vi "prelim_per_setup.vi"(8 "error in":errorcluster, 11 "reference cluster":T1) -> (0 "error out":errorcluster, 3 "reference cluster":T1)   [LabVIEW 2016]
uses:
  Type Definitions/reference_cluster.ctl
  Type Definitions/vars_settings.ctl
  Type Definitions/stim_type.ctl
  Type Definitions/backlight_type.ctl
  Type Definitions/vars_runtime.ctl
  Type Definitions/data.ctl
  Type Definitions/notifier_elements_GUI.ctl
  Type Definitions/notifier_elements_DAQ.ctl
  Type Definitions/notifier_elements_write.ctl
  Type Definitions/control_references.ctl
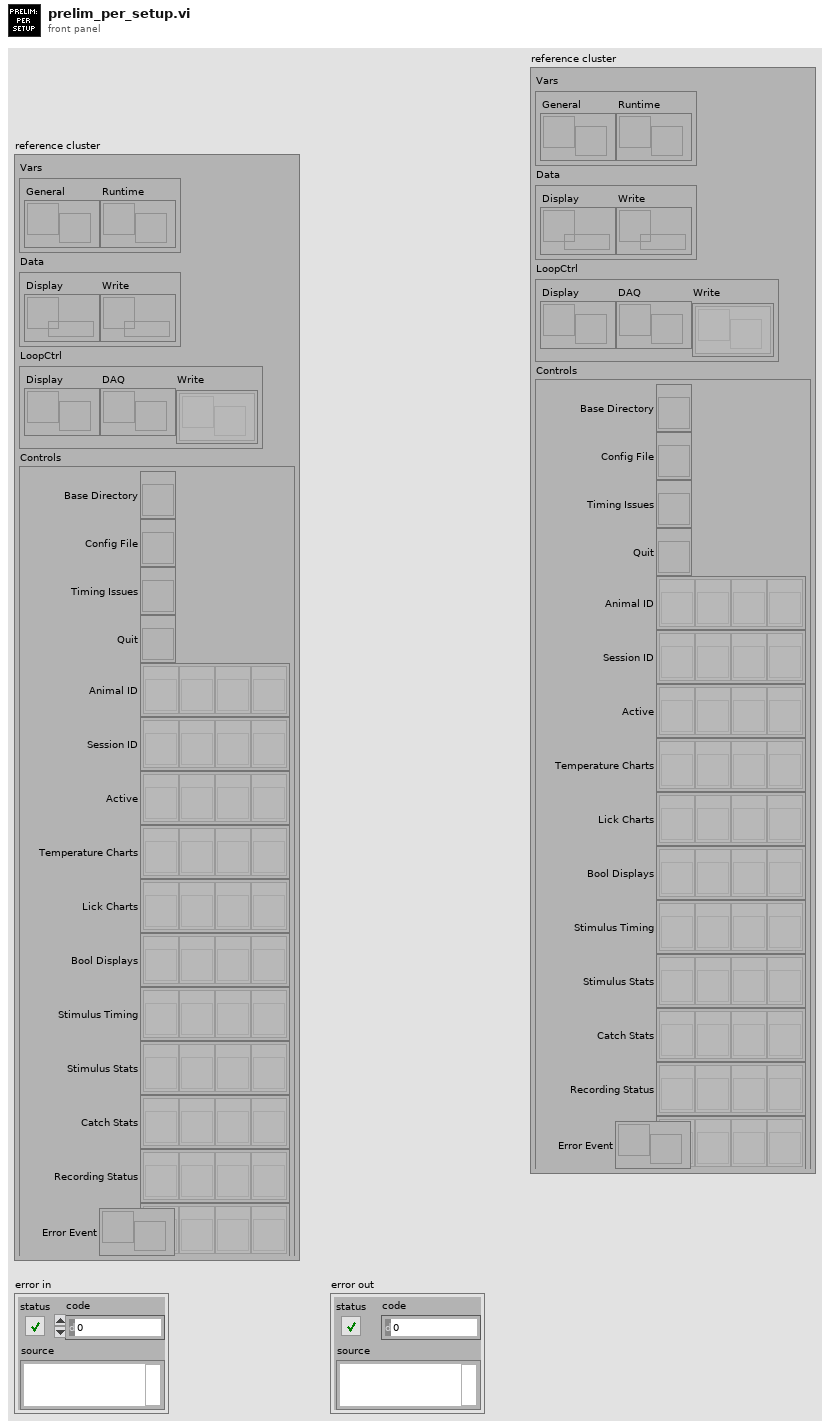
[diagram p1: front panel]
types:
  T1 = typedef "reference_cluster.ctl" = cluster{"Vars":cluster{"General":refnum<notifier>, "Runtime":refnum<notifier>}, "Data":cluster{"Display":refnum<queue>, "Write":refnum<queue>}, "LoopCtrl":cluster{"Display":refnum<notifier>, "DAQ":refnum<notifier>, "Write":refnum<notifier>[]}, "Controls":T2, "Error Event":refnum<user-event>}
  T2 = typedef "control_references.ctl" = cluster{"Base Directory":refnum<vi>, "Config File":refnum<vi>, "Timing Issues":refnum<vi>, "Quit":refnum<vi>, "Animal ID":refnum<vi>[], "Session ID":refnum<vi>[], "Active":refnum<vi>[], "Temperature Charts":refnum<vi>[], "Lick Charts":refnum<vi>[], "Bool Displays":refnum<vi>[], "Stimulus Timing":refnum<vi>[], "Stimulus Stats":refnum<vi>[], "Catch Stats":refnum<vi>[], "Recording Status":refnum<vi>[], "Pairing":refnum<vi>[]}
  T3 = typedef "vars_settings.ctl" = cluster{"base directory":path, "data directory":path, "active":bool, "running":bool, "pairing":bool, "clean tubes":bool, "animal ID":u16, "session ID":u16, "base temp":dbl, "d wait min":u16, "d wait max":u16, "d timeout":u16, "d timeout catch":u16, "d penalty":u16, "d reward":u16, "n reward":u16, "idx stim":u16, "timeout win":u16, "lick win":i32[], "stim type":T4[], "stim dur":u16[], "stim amp":dbl[], "stim freq":u16[], "stim ramp":u16[], "stim catch":u8[], "pairing delay":i16[], "square dur":u16[], "square delay":i16[], "square freq":u8[], "square dc":u8[], "stim shape":dbl[][], "square shape":bool[][], "backlight type":T5, "backlight freq":u16, "dStimOne dur":u16[], "dStimOne delay":i16[], "dStimTwo dur":u16[], "dStimTwo delay":i16[]}
  T4 = typedef "stim_type.ctl" = enum16{"pulse", "vibration", "square", "sine"}
  T5 = typedef "backlight_type.ctl" = enum16{"none", "random", "regular"}
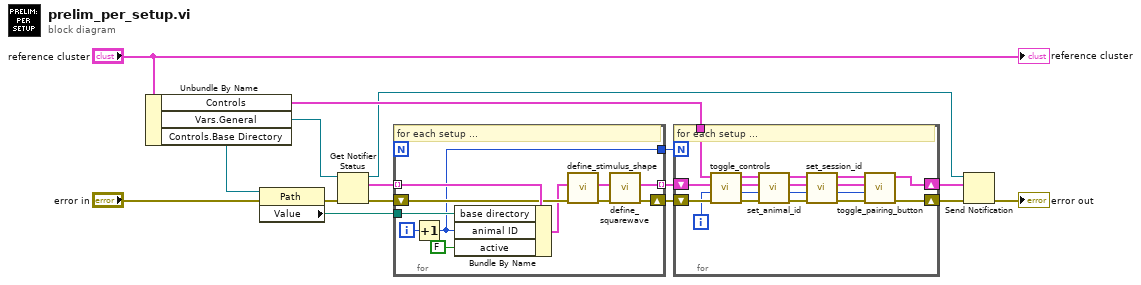
[diagram p0: block diagram]
diagram:
  n1 = Unbundle By Name("reference cluster") -> ("Controls"=w14:T2, "Vars.General"=w5:refnum<notifier>, "Controls.Base Directory"=w4:refnum<vi>)
  n2 = property class="Path"(reference=w4, error in="error in") -> (error out=w2:errorcluster, "Value"=w1:path)  [unwired: 1 out]
  n3 = Get Notifier Status(notifier=w5, error in (no error)=w2) -> (notifier out=w11:refnum<notifier>, current notification=w7:T3[], error out=w6:errorcluster)  [unwired: 2 out]
  n4 = for {
    shift-right: [w17] -> w12
    shift-left: w6 -> [w25]
    tunnel: w7 -> [w27] mode=indexing
    tunnel: w1 -> [w26]
    tunnel: [w22] -> w8
    tunnel: [w18] -> w10 mode=indexing
    i -> [w23]
    # "for each setup ..."
    n5 = Increment(x=w23) -> (x+1=w22:i32)
    n6 = Bundle By Name(cluster=w27, "base directory"=w26, "animal ID"=w22, "active"=FALSE) -> (w24:T3)
    n7 = call "define_stimulus_shape.vi"("error in"=w25, "input cluster"=w24) -> ("error out"=w19:errorcluster, "output cluster"=w20:T3)  [unwired: 8 in]
    n8 = call "define_squarewave.vi"("input cluster"=w20, "error in"=w19) -> ("output cluster"=w18:T3, "error out"=w17:errorcluster)  [unwired: 7 in]
  }
  n9 = for {
    N: w8 -> [_]
    shift-right: [w31] -> w9
    shift-left: w12 -> [w37]
    tunnel: w14 -> [w34]
    shift-right: [w32] -> w13
    shift-left: w10 -> [w35]
    i -> [w36]
    # "for each setup ..."
    n10 = call "toggle_controls.vi"("error in"=w37, "setup ID"=w36, "vars general in"=w35, "control cluster in"=w34) -> ("error out"=w41:errorcluster, "setup ID"=w38:i32, "vars general out"=w39:T3[], "control cluster out"=w40:T2)  [unwired: 4 in]
    n11 = call "set_animal_id.vi"("error in"=w41, "setup ID"=w38, "settings array in"=w39, "control cluster in"=w40) -> ("error out"=w45:errorcluster, "setup ID"=w44:u16, "settings array out"=w43:T3[], "control cluster out"=w42:T2)  [unwired: 2 in]
    n12 = call "set_session_id.vi"("control cluster in"=w42, "settings in"=w43, "setup ID"=w44, "error in"=w45) -> ("control cluster out"=w30:T2, "settings out"=w29:T3[], "Setup ID"=w28:i32, "error out"=w33:errorcluster)  [unwired: 3 in]
    n13 = call "toggle_pairing_button.vi"("error in"=w33, "Setup ID"=w28, "settings in"=w29, "control cluster in"=w30) -> ("error out"=w31:errorcluster, "settings out"=w32:T3[])  [unwired: 6 in]
  }
  n14 = Send Notification(notification=w13, notifier=w11, error in (no error)=w9) -> (error out=→"error out":errorcluster)  [unwired: 1 out]
  "reference cluster" <- "reference cluster"
